vi "RPI.SenseHat.Actor Launcher.vi"(8 "error in (no error)":errorcluster) -> (0 "error out":errorcluster, 3 "RPI.SenseHat Enqueuer":refnum<class "Message Enqueuer.lvclass">)   [LabVIEW 2020, in "RPI.SenseHat.Actor.lvlib"]
uses:
  RPI.SenseHat.Actor.lvlib
  <vilib>/ActorFramework/Message Enqueuer/Message Enqueuer.lvclass
  RPI.SenseHat.Actor/RPI.SenseHat.Actor.lvclass
  C:/Program Files (x86)/National Instruments/LabVIEW 2020/vi.lib/ActorFramework/Actor/Actor.lvclass
  <vilib>/ActorFramework/Actor/Actor.lvclass
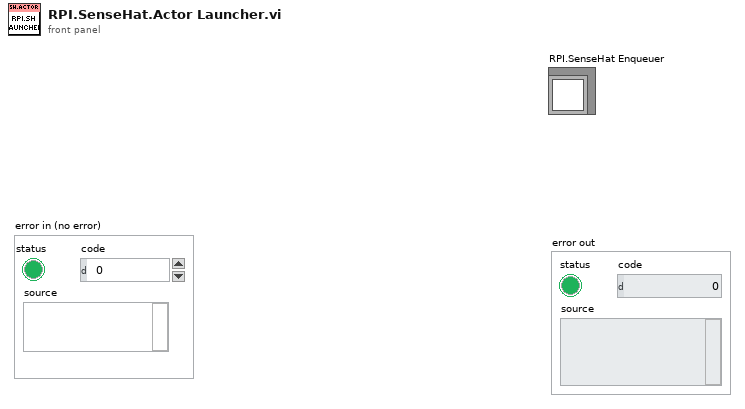
[diagram p1: front panel]
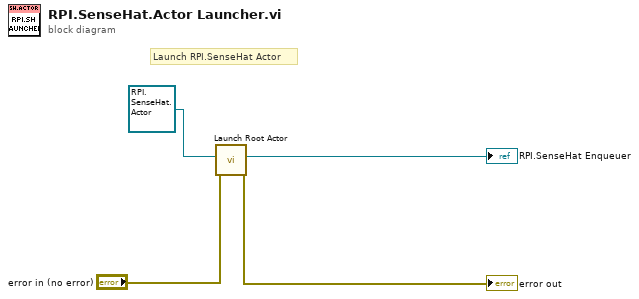
[diagram p0: block diagram]
diagram:
  # "Launch RPI.SenseHat Actor"
  n1 = call <vilib>:"Launch Root Actor.vi"("error in (no error)"="error in (no error)", "Actor"=refnum<class "RPI.SenseHat.Actor.lvclass"> refnum ("RPI.SenseHat.Actor.lvlib:RPI.SenseHat.Actor.lvclass")) -> ("error out"=→"error out":errorcluster, "Actor's Enqueuer"=→"RPI.SenseHat Enqueuer":refnum<class "Message Enqueuer.lvclass">)  [unwired: 8 in]
